vi "Read PNAMES.vi"(11 "Lump DATA IN":u8[](array[numeric])) -> (3 "PNAMES Array":string[](array[string]))   [LabVIEW 2017]
uses:
  <vilib>/Utility/error.llb/Search and Replace Pattern.vi
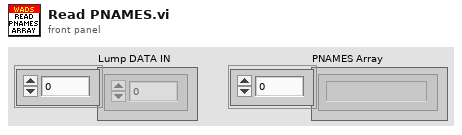
[diagram p1: front panel]
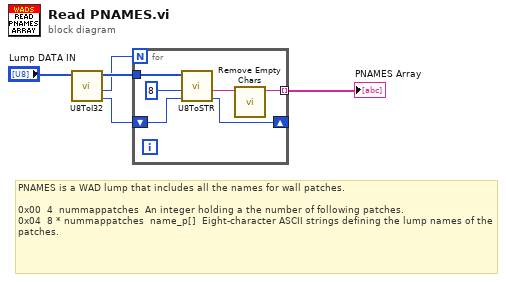
[diagram p0: block diagram]
diagram:
  # "PNAMES is a WAD lump that includes all the names for wall patches.\n\n0x00 \t4 \tnummappatches \tAn integer holding a the number of following patches.\n0x04 \t8 * nummappatches \tname_p[] \tEight-character ASCII strings defining the lump names of the patches."
  n1 = call "U8ToI32.vi"("Input U8 Array"="Lump DATA IN") -> ("Index+4"=w4:u32, "Output I32"=w2:i32, "Output U8 Array"=w3:u8[])  [unwired: 4 in]
  n2 = for {
    N: w2 -> [_]
    tunnel: w3 -> [w10]
    shift-right: [w8] -> _
    shift-left: w4 -> [w9]
    tunnel: [w6] -> w5 mode=indexing
    n3 = call "U8ToSTR.vi"("Index"=w9, "Count"=8, "Input U8 Array"=w10) -> ("Index+Count"=w8:u32, "Output String"=w7:string)  [unwired: 2 in, 1 out]
    n4 = call "Remove Empty Chars.vi"("String with \\00"=w7) -> ("String without \\00"=w6:string)  [unwired: 10 in]
  }
  "PNAMES Array" <- w5
